vi "MotorDualDirection.vi"() -> ()   [LabVIEW 2014]
panel:
  out "Motor Terminal -":bool
  out "Motor Terminal +":bool
  out "Reverse":bool
  in  "Forward":bool
  in  "On/Off":bool
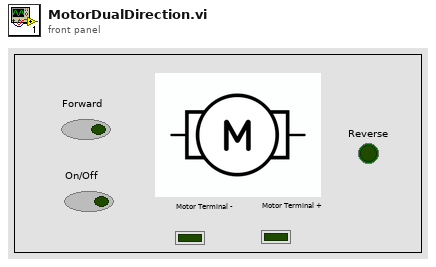
[diagram p1: front panel]
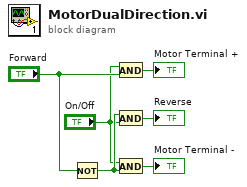
[diagram p0: block diagram]
diagram:
  n1 = Not(x="Forward") -> (.not. x?=w2:bool)
  n2 = And(x="On/Off", y="Forward") -> (x .and. y?=→"Motor Terminal +":bool)
  n3 = And(x=w2, y="On/Off") -> (x .and. y?=→"Reverse":bool)
  n4 = And(x="On/Off", y=w2) -> (x .and. y?=→"Motor Terminal -":bool)
